vi "运维调试_五参数.vi"() -> ()   [LabVIEW 2016, in "斯坦道仪器.lvlib"]
uses:
  <vilib>/Utility/miscctls.llb/LVPointTypeDef.ctl
  PLC/PLC.lvlib
panel:
  in  "打开串口":bool
  in  "释放串口":bool
  out "数值 2":i32
  out "数值":i32
  in  "手动通电":bool
  out "多参数横条运行状态":T1(xcontrol)
  in  "数据区":i32(listbox)
  in  "探头选择":u16(ring)=9 items=["氨氮"=3, "水温"=9, "pH值"=10, "溶解氧"=11, "电导率"=12, "浊度"=13, "叶绿素a"=14, "藻密度"=15, "蓝绿藻"=16, "氧化还原电位"=17, "溶解氧%"=18, "盐度"=19]
  in  "测量数据区读取":bool
  in  "测量数据区":i32(listbox)
  in  "状态告警区读取":bool
  in  "状态告警区":i32(listbox)
  in  "自动校准":bool
  in  "读取KB":bool
  in  "写入KB":bool
  out "B":dbl caption="校准值B:"
  out "K":dbl caption="校准值K:"
  in  "校准区探头选择":u16(ring)=9 items=["氨氮"=3, "水温"=9, "pH值"=10, "溶解氧"=11, "电导率"=12, "浊度"=13, "叶绿素a"=14, "藻密度"=15, "蓝绿藻"=16, "氧化还原电位"=17, "溶解氧%"=18, "盐度"=19]
  in  "停止测量(单探)":bool
  in  "启动测量(单探)":bool
  in  "控制命令区探头选择":u16(ring)=9 items=["氨氮"=3, "水温"=9, "pH值"=10, "溶解氧"=11, "电导率"=12, "浊度"=13, "叶绿素a"=14, "藻密度"=15, "蓝绿藻"=16, "氧化还原电位"=17, "溶解氧%"=18, "盐度"=19]
  in  "同步时间":bool
  in  "初始化(清洗)":bool
  in  "停止测量(全部)":bool
  in  "启动测量(全部)":bool
  in  "关键参数区读取":bool
  in  "关键参数区":i32(listbox)
  in  "传感器参数读取":bool
  in  "传感器区":i32(listbox)
  in  "返回":bool
  in  "设置":bool
  out "运行状态":string
  out "开机状态":bool
  in  "停止":bool
  in  "手动启动":bool
  out "集成报警信息":string
  # "控制命令区"
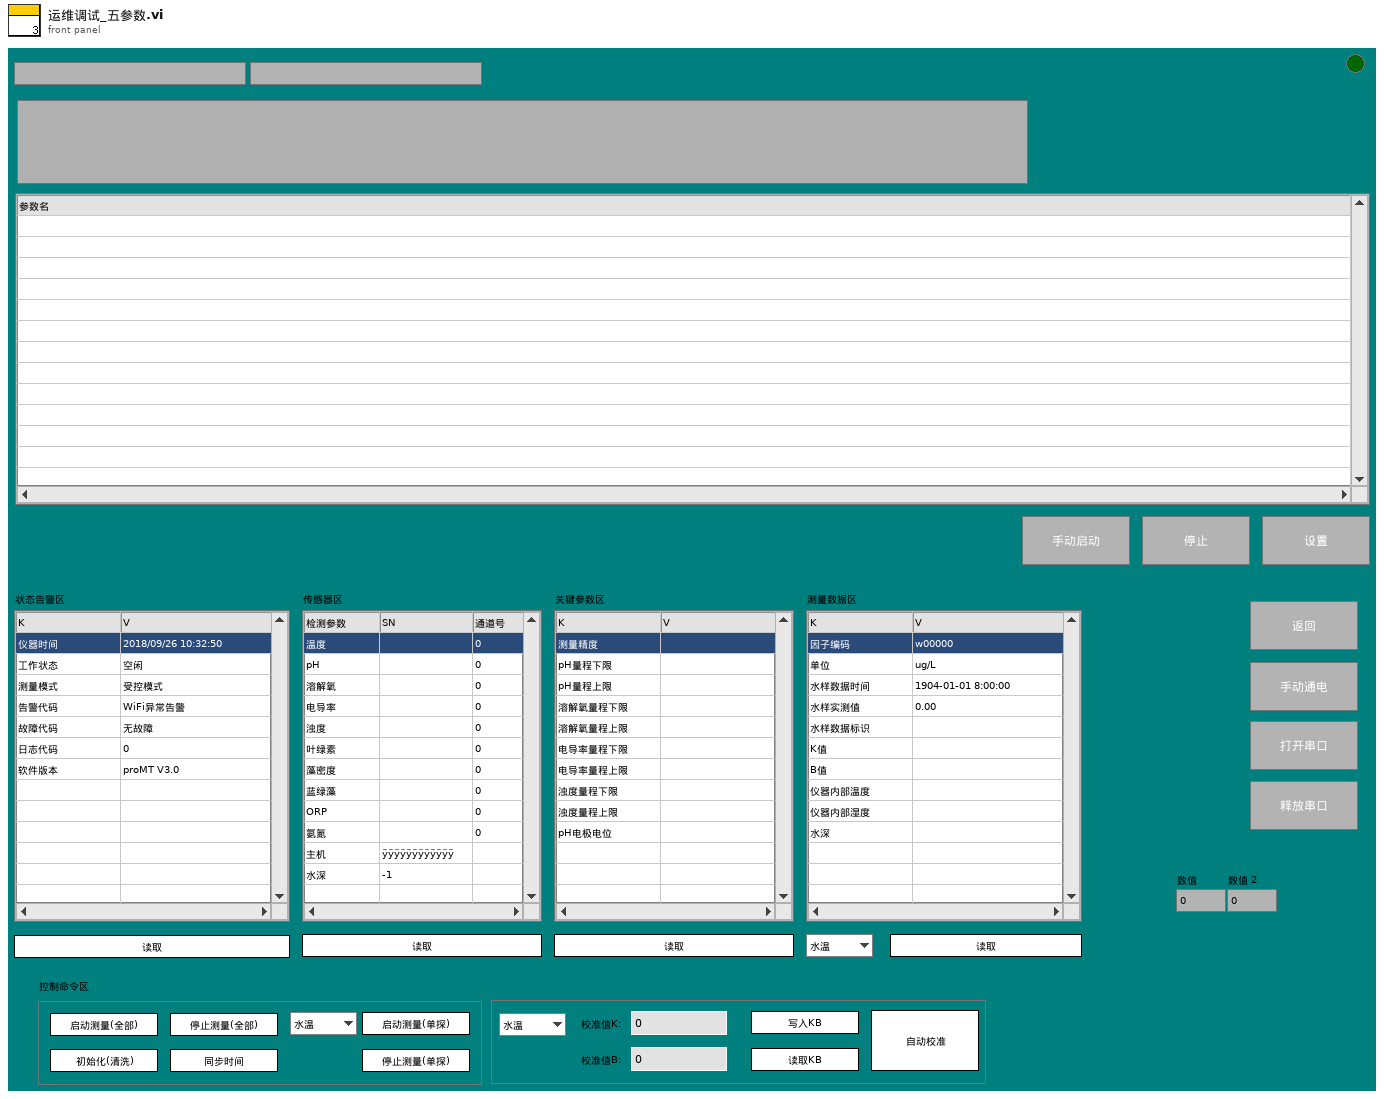
[diagram p1: front panel]
types:
  T1 = cluster{"系统时间":timestamp, "工作状态":u16, "测量模式":u16, "告警代码":enum16{"无告警", "缺试剂告警", "缺水样告警", "缺蒸馏水告警", "缺标液告警", "仪表漏液告警", "标定异常告警", "超量程告警", "加热异常", "低试剂预警", "超上限告警", "超下限告警", "仪表内部其他异常", "滴定异常告警", "电极异常告警", "量程切换告警", "参数设置告警", "PH电极电位异常", "电导率电极异常", "浊度光度异常", "溶解氧电极异常", "溶解氧光强异常", "温度异常告警", "PH异常告警", "溶解氧异常告警", "电导率异常告警", "浊度异常告警", "叶绿素异常告警", "藻密度异常告警", "蓝绿藻异常告警", "ORP异常告警", "氨氮异常告警", "清洁刷异常告警", "SD卡异常告警", "蓝牙异常告警", "Wifi异常告警", "流程异常告警"}, "故障代码":enum16{"无故障", "电机故障", "温度故障", "通讯故障", "滴定故障"}, "日志代码":u16, "软件版本":string}
  T2 = typedef "LVPointTypeDef.ctl" = cluster{"Horizontal":i16, "Vertical":i16}
  T3 = cluster{"时间标识":timestamp, "设备":string, "日志信息":string}
  T4 = enum16{"无告警", "缺试剂告警", "缺水样告警", "缺蒸馏水告警", "缺标液告警", "仪表漏液告警", "标定异常告警", "超量程告警", "加热异常", "低试剂预警", "超上限告警", "超下限告警", "仪表内部其他异常", "滴定异常告警", "电极异常告警", "量程切换告警", "参数设置告警", "PH电极电位异常", "电导率电极异常", "浊度光度异常", "溶解氧电极异常", "溶解氧光强异常", "温度异常告警", "PH异常告警", "溶解氧异常告警", "电导率异常告警", "浊度异常告警", "叶绿素异常告警", "藻密度异常告警", "蓝绿藻异常告警", "ORP异常告警", "氨氮异常告警", "清洁刷异常告警", "SD卡异常告警", "蓝牙异常告警", "Wifi异常告警", "流程异常告警"}
  T5 = cluster{"WORD[0]":u16, "WORD[1]":u16, "WORD[2]":u16, "WORD[3]":u16, "WORD[4]":u16, "WORD[5]":u16, "WORD[6]":u16, "WORD[7]":u16, "WORD[8]":u16, "WORD[9]":u16}
  T6 = cluster{"因子编码":string, "单位":string, "标样参考值":sgl, "水样数据时间":timestamp, "水样实测值":sgl, "水样数据标识":string, "K":sgl, "B":sgl, "T":sgl, "H":sgl, "水深":sgl}
  T7 = enum8{"Enabled", "Disabled", "Disabled and Grayed Out"}
  T8 = cluster{"测量模式":enum16{"待机", "水样测试", "标样核查", "零点核查", "跨度核查", "空白测试", "平行样测试", "加标回收", "空白校准", "标样校准", "初始化（清洗）"}, "数据标记表":string, "测量时间":dbl}
  T9 = cluster{"starting address":u16, "holding register value":u16}
  T10 = enum16{"idle", "init", "读状态", "读参数", "多个写入", "单个写入", "线圈写入"}
  T11 = enum32{"Bad", "Idle", "Run top level", "Running"}
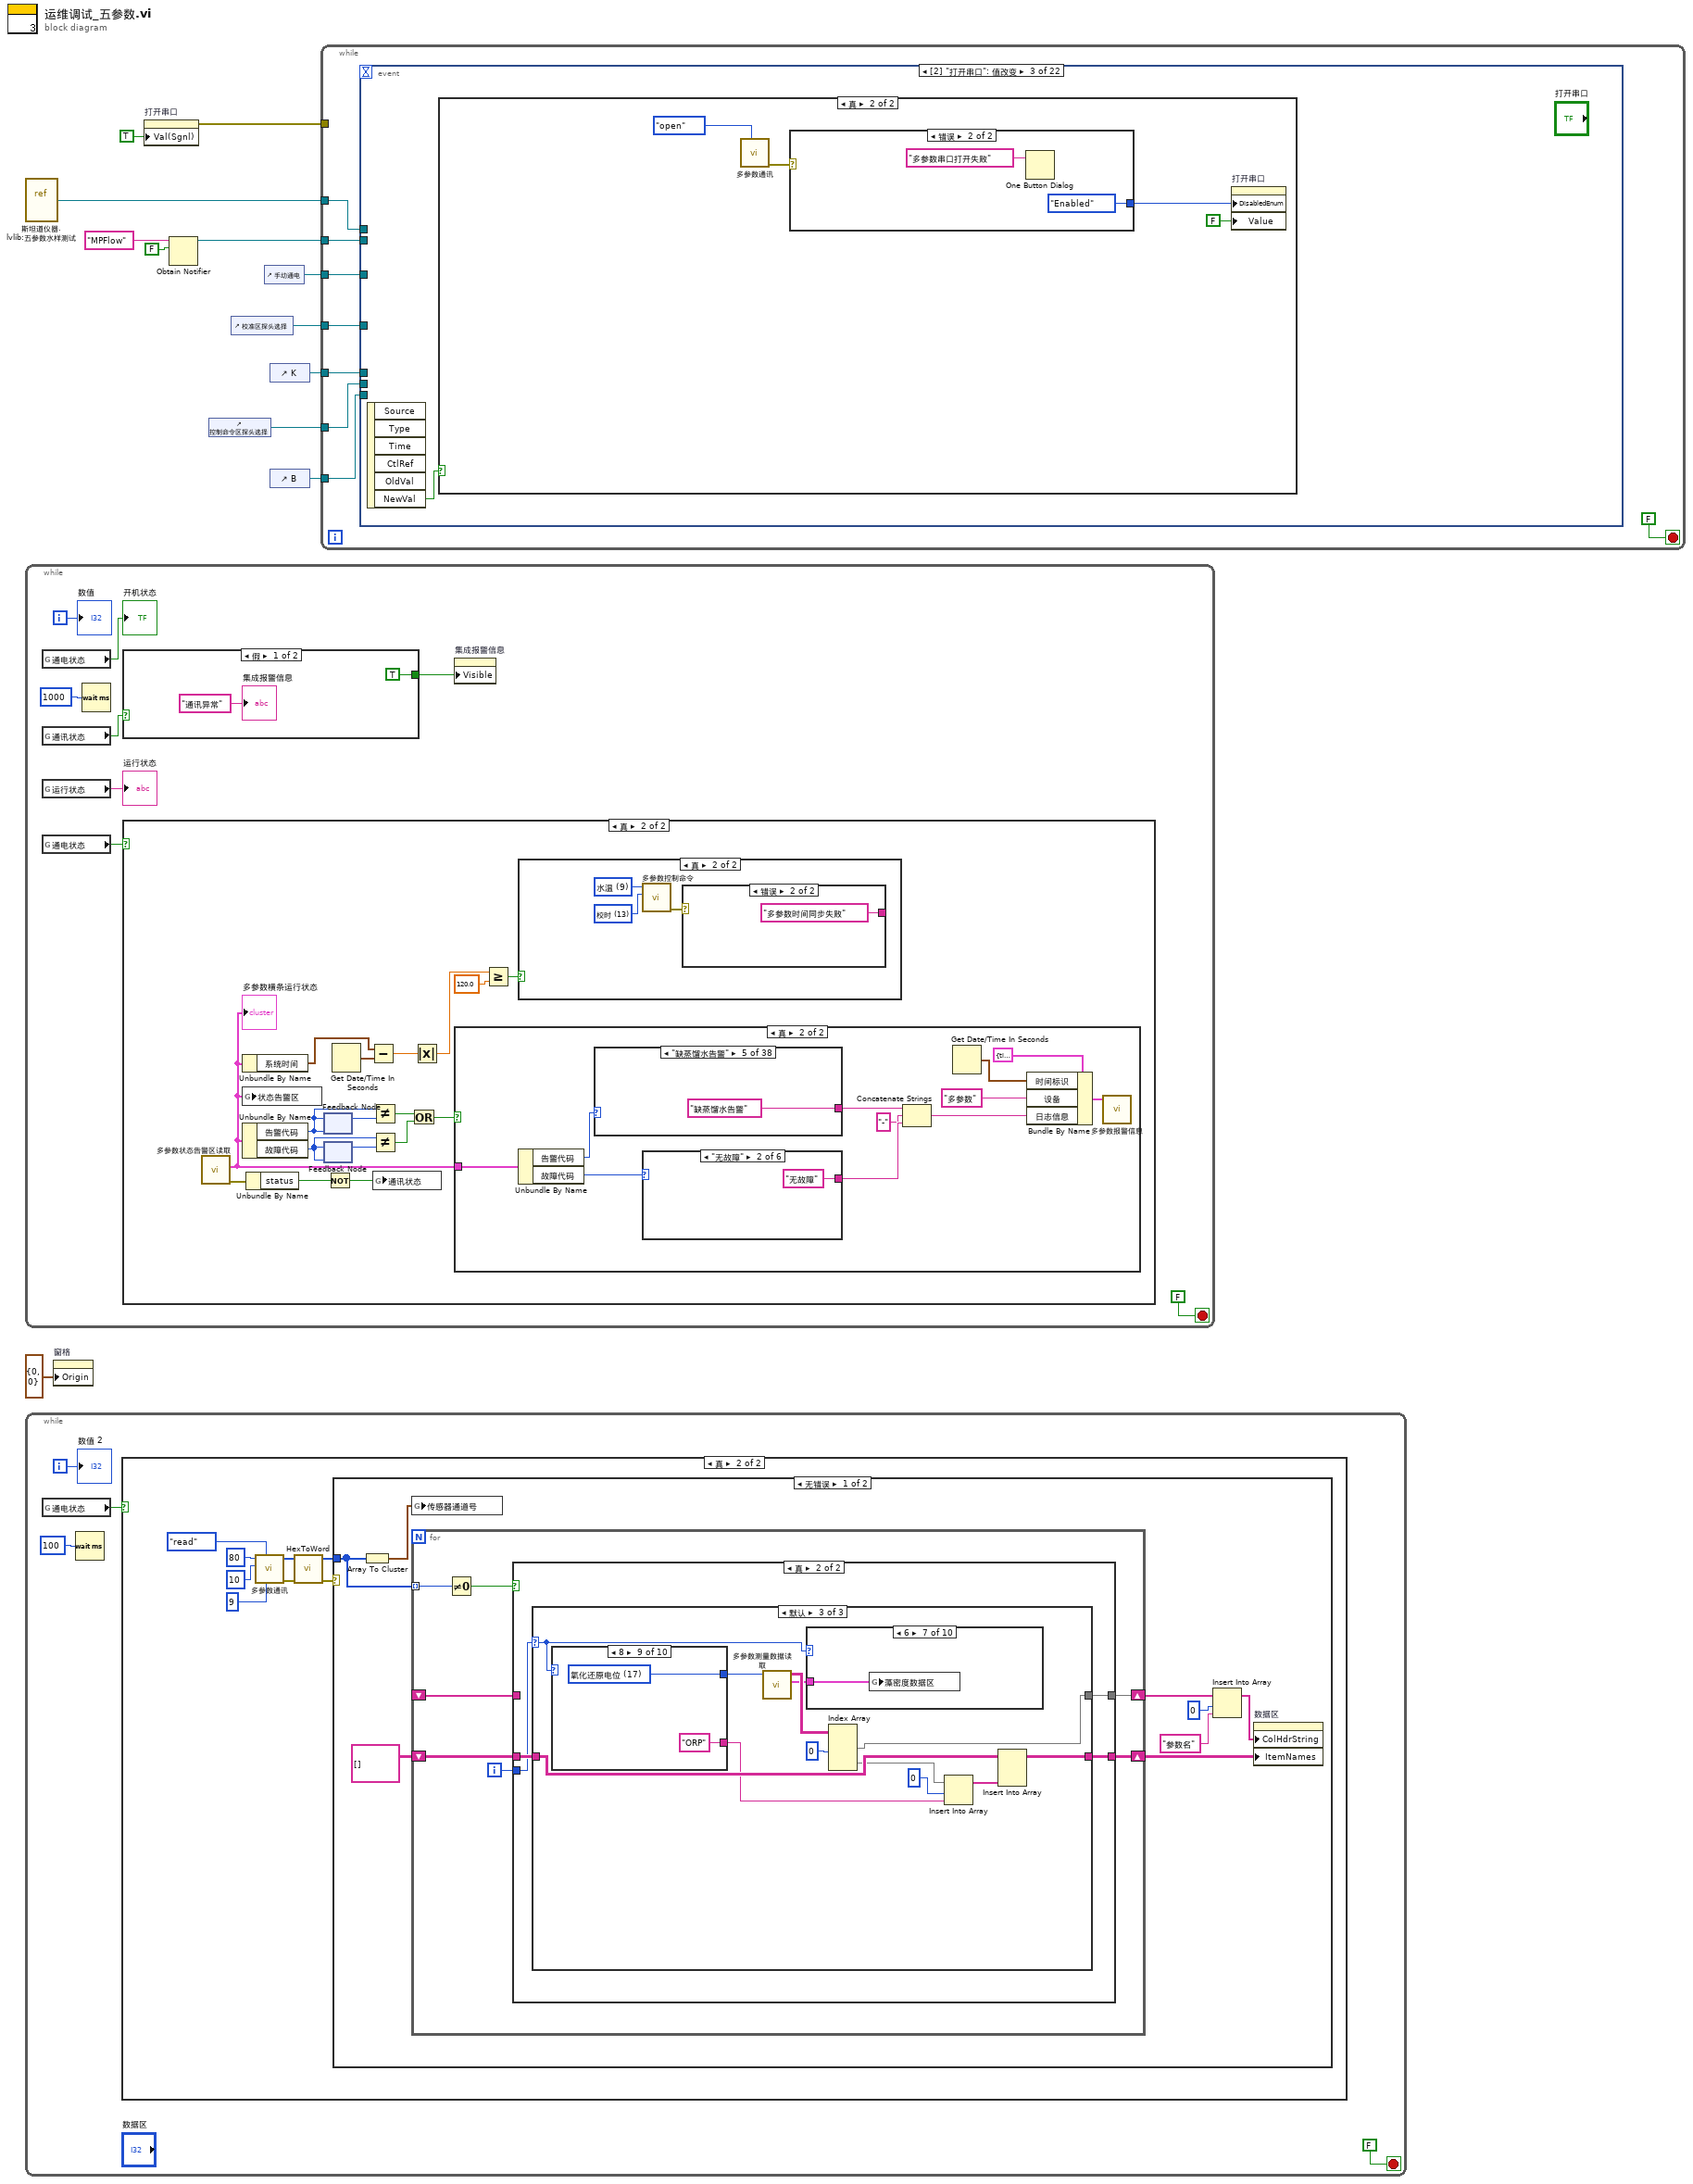
[diagram p0: block diagram]
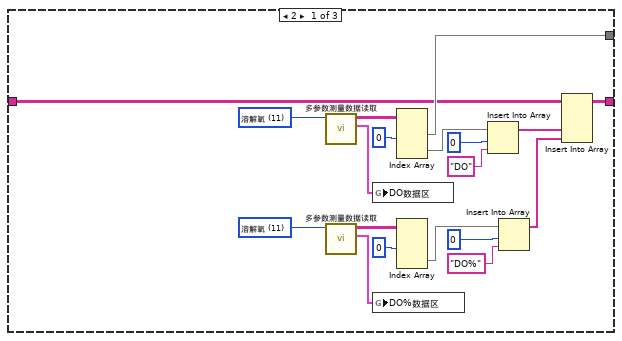
[diagram p4: hidden frame]
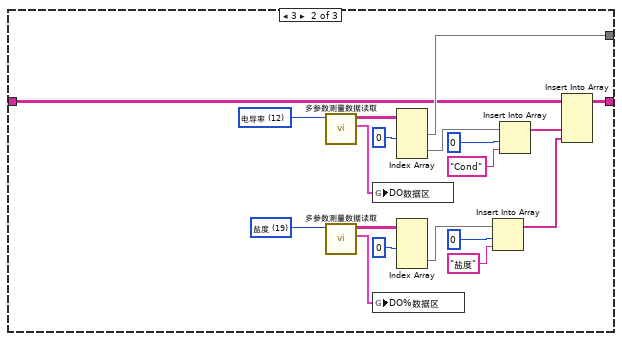
[diagram p5: hidden frame]
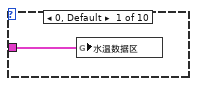
[diagram p6: hidden frame]
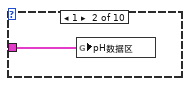
[diagram p7: hidden frame]
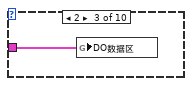
[diagram p8: hidden frame]
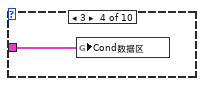
[diagram p9: hidden frame]
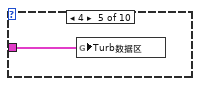
[diagram p10: hidden frame]
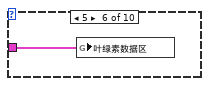
[diagram p11: hidden frame]
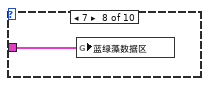
[diagram p12: hidden frame]
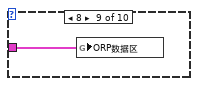
[diagram p13: hidden frame]
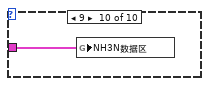
[diagram p14: hidden frame]
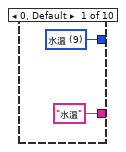
[diagram p15: hidden frame]
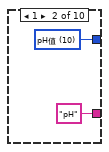
[diagram p16: hidden frame]
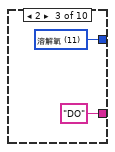
[diagram p17: hidden frame]
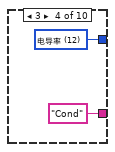
[diagram p18: hidden frame]
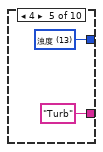
[diagram p19: hidden frame]
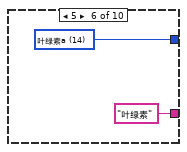
[diagram p20: hidden frame]
diagram:
  n1 = vi-ref "斯坦道仪器.lvlib:五参数水样测试.vi"() -> (w9:refnum<vi>)
  n2 = while {
    i -> [w13]
    stop <- FALSE stop-if-true
    n3 = global read "多参数全局变量.vi" "通电状态"() -> (→"开机状态":bool)
    n4 = global read "多参数全局变量.vi" "通讯状态"() -> (w18:bool)
    n5 = global read "多参数全局变量.vi" "运行状态"() -> (→"运行状态":string)
    n6 = global read "多参数全局变量.vi" "通电状态"() -> (w14:bool)
    n7 = Wait (ms)(milliseconds to wait=u32 1000 ("等待时间（毫秒）")) -> ()  [unwired: 1 out]
    n8 = case shown="假" w18 {
      tunnel: [TRUE ("可见") _] -> w17
      frame False {
        "集成报警信息" <- "通讯异常" ("集成报警信息")
      }
      frame True {
      }
    }
    n9 = case shown="真" w14 {
      frame False {
      }
      frame True {
        n10 = call "多参数状态告警区读取.vi"() -> ("error out"=w30:errorcluster, "状态告警块"=w27:T1)  [unwired: 9 in, 1 out]
        "多参数横条运行状态" <- w27
        n11 = Unbundle By Name(w27) -> ("系统时间"=w26:timestamp)
        n12 = global write "多参数全局变量.vi" "状态告警区"(w27) -> ()
        n13 = Unbundle By Name(w27) -> ("告警代码"=w36:T4, "故障代码"=w34:enum16{"无故障", "电机故障", "温度故障", "通讯故障", "滴定故障"})
        n14 = Unbundle By Name(w30) -> ("status"=w29:bool)
        n15 = feedback #1(w36) -> (w37:T4)
        n16 = feedback-in #1(w36) -> ()
        n17 = feedback #2(w34) -> (w35:enum16{"无故障", "电机故障", "温度故障", "通讯故障", "滴定故障"})
        n18 = feedback-in #2(w34) -> ()
        n19 = Not(x=w29) -> (.not. x?=w28:bool)
        n20 = Get Date/Time In Seconds() -> (seconds since 1Jan1904=w25:timestamp)
        n21 = Subtract(x=w26, y=w25) -> (x-y=w24:dbl)
        n22 = Not Equal?(x=w36, y=w37) -> (x != y?=w32:bool)
        n23 = Not Equal?(x=w34, y=w35) -> (x != y?=w33:bool)
        n24 = global write "多参数全局变量.vi" "通讯状态"(w28) -> ()
        n25 = Or(x=w32, y=w33) -> (x .or. y?=w31:bool)
        n26 = Absolute Value(x=w24) -> (abs(x)=w23:dbl)
        n27 = case shown="真" w31 {
          tunnel: w27 -> [_ w53]
          frame False {
          }
          frame True {
            n28 = Unbundle By Name(w53) -> ("告警代码"=w52:T4, "故障代码"=w51:enum16{"无故障", "电机故障", "温度故障", "通讯故障", "滴定故障"})
            n29 = case shown="\"缺蒸馏水告警\"" w52 {
              selector: w52 -> [w64 _ _ _ _ _ _ _ _ _ _ _ _ _ _ _ _ _ _ _ _ _ _ _ _ _ _ _ _ _ _ _ _ _ _ _ _ _]
              tunnel: [w63 "无告警" "缺试剂告警" "缺水样告警" "缺蒸馏水告警" "缺标液告警" "仪表漏液告警" "标定异常告警" "超量程告警" "加热异常" "低试剂预警" "超上限告警" "超下限告警" "仪表内部其他异常" "滴定异常告警" "电极异常告警" "量程切换告警" "参数设置告警" "PH电极电位异常" "电导率电极异常" "浊度光度异常" "溶解氧电极异常" "溶解氧光强异常" "温度异常告警" "PH异常告警" "溶解氧异常告警" "电导率异常告警" "浊度异常告警" "叶绿素异常告警" "藻密度异常告警" "蓝绿藻异常告警" "ORP异常告警" "氨氮异常告警" "清洁刷异常告警" "SD卡异常告警" "蓝牙异常告警" "WiFi异常告警" "流程异常告警"] -> w50
              frame Default {
                n30 = Format Into String(format string="%d" ("格式字符串"), initial string="未知" ("工作状态"), w64) -> (resulting string=w63:string)  [unwired: 1 in, 1 out]
              }
              frame "无告警" {
              }
              frame "缺试剂告警" {
              }
              frame "缺水样告警" {
              }
              frame "缺蒸馏水告警" {
              }
              frame "缺标液告警" {
              }
              frame "仪表漏液告警" {
              }
              frame "标定异常告警" {
              }
              frame "超量程告警" {
              }
              frame "加热异常" {
              }
              frame "低试剂预警" {
              }
              frame "超上限告警" {
              }
              frame "超下限告警" {
              }
              frame "仪表内部其他异常" {
              }
              frame "滴定异常告警" {
              }
              frame "电极异常告警" {
              }
              frame "量程切换告警" {
              }
              frame "参数设置告警" {
              }
              frame "PH电极电位异常" {
              }
              frame "电导率电极异常" {
              }
              frame "浊度光度异常" {
              }
              frame "溶解氧电极异常" {
              }
              frame "溶解氧光强异常" {
              }
              frame "温度异常告警" {
              }
              frame "PH异常告警" {
              }
              frame "溶解氧异常告警" {
              }
              frame "电导率异常告警" {
              }
              frame "浊度异常告警" {
              }
              frame "叶绿素异常告警" {
              }
              frame "藻密度异常告警" {
              }
              frame "蓝绿藻异常告警" {
              }
              frame "ORP异常告警" {
              }
              frame "氨氮异常告警" {
              }
              frame "清洁刷异常告警" {
              }
              frame "SD卡异常告警" {
              }
              frame "蓝牙异常告警" {
              }
              frame "Wifi异常告警" {
              }
              frame "流程异常告警" {
              }
            }
            n31 = case shown="\"无故障\"" w51 {
              selector: w51 -> [w55 _ _ _ _ _]
              tunnel: [w54 "无故障" "电机故障" "温度故障" "通讯故障" "滴定故障"] -> w49
              frame Default {
                n32 = Format Into String(format string="%d" ("格式字符串"), initial string="未知" ("工作状态"), w55) -> (resulting string=w54:string)  [unwired: 1 in, 1 out]
              }
              frame "无故障" {
              }
              frame "电机故障" {
              }
              frame "温度故障" {
              }
              frame "通讯故障" {
              }
              frame "滴定故障" {
              }
            }
            n33 = Concatenate Strings(w50, "-" ("字符串"), w49) -> (w45:string)
            n34 = Get Date/Time In Seconds() -> (seconds since 1Jan1904=w44:timestamp)
            n35 = Bundle By Name(cluster=T3 {"时间标识"=timestamp(0 s since 1904-01-01), "设备"="", "日志信息"=""} ("data in"), "时间标识"=w44, "设备"="多参数", "日志信息"=w45) -> (w46:T3)
            n36 = call "多参数报警信息.vi"("data in"=w46) -> ()  [unwired: 10 in, 1 out]
          }
        }
        n37 = Greater Or Equal?(x=w23, y=120.0) -> (x >= y?=w22:bool)
        n38 = case shown="真" w22 {
          frame False {
          }
          frame True {
            w38 = u16 13 items=["启动测量（全部）"=1, "初始化（清洗）"=10, "停止测量（全部）"=11, "校时"=13, "启动测量（单个传感器）"=19, "停止测量（单个传感器）"=20] ("控制命令")
            w39 = u16 9 items=["氨氮"=3, "水温"=9, "pH值"=10, "溶解氧"=11, "电导率"=12, "浊度"=13, "叶绿素a"=14, "藻密度"=15, "蓝绿藻"=16, "氧化还原电位"=17, "溶解氧%"=18, "盐度"=19] ("站号")
            n39 = call "多参数控制命令.vi"("控制命令"=w38, "站号"=w39) -> ("error out"=w40:errorcluster)  [unwired: 9 in]
            n40 = case shown="错误" w40 {
              tunnel: ["多参数时间同步成功" ("消息") "多参数时间同步失败" ("消息")] -> _
              frame No Error {
              }
              frame Error {
              }
            }
          }
        }
      }
    }
    n41 = property on="集成报警信息" class="Str"("Visible"=w17) -> ()  [unwired: 2 in, 2 out]
    "数值" <- w13
  }
  n42 = while {
    i -> [w106]
    stop <- FALSE stop-if-true
    n43 = global read "多参数全局变量.vi" "通电状态"() -> (w107:bool)
    n44 = Wait (ms)(milliseconds to wait=u32 100 ("等待时间（毫秒）")) -> ()  [unwired: 1 out]
    n45 = case shown="真" w107 {
      frame False {
      }
      frame True {
        n46 = call "多参数通讯.vi"("Slave ID"=u8 9, "STEP"=enum16{"open", "read", "write", "close"}."read", "quantity"=u16 10, "starting address"=u16 80) -> ("error out"=w112:errorcluster, "Registers"=w113:u16[])  [unwired: 5 in, 1 out]
        n47 = call "HexToWord.vi"("数组"=w113) -> ("WORD"=w116:u16[])  [unwired: 10 in]
        n48 = case shown="无错误" w112 {
          tunnel: w116 -> [w117 _]
          frame No Error {
            n49 = Array To Cluster(array=w117) -> (cluster=w118:T5)
            n50 = global write "多参数全局变量.vi" "传感器通道号"(w118) -> ()
            n51 = for {
              tunnel: w117 -> [w130] mode=indexing
              shift-right: [w128] -> w122
              shift-left: _ -> [w127]
              shift-right: [w125] -> w123
              shift-left: string[][] [] ("子数组") -> [w126]
              i -> [w131]
              n52 = Not Equal To 0?(x=w130) -> (x != 0?=w129:bool)
              n53 = case shown="真" w129 {
                tunnel: w131 -> [_ w134]
                tunnel: [w133 w137] -> w128
                tunnel: w127 -> [w133 _]
                tunnel: w126 -> [w132 w136]
                tunnel: [w132 w135] -> w125
                frame False {
                }
                frame True {
                  n54 = case shown="默认" w134 {
                    selector: w134 -> [_ _ w176]
                    tunnel: [w146 w165 w184] -> w137
                    tunnel: w136 -> [w142 w161 w183]
                    tunnel: [w145 w164 w182] -> w135
                    frame 2 {
                      w140 = u16 11 items=["氨氮"=3, "水温"=9, "pH值"=10, "溶解氧"=11, "电导率"=12, "浊度"=13, "叶绿素a"=14, "藻密度"=15, "蓝绿藻"=16, "氧化还原电位"=17, "溶解氧%"=18, "盐度"=19] ("探头选择")
                      w141 = u16 11 items=["氨氮"=3, "水温"=9, "pH值"=10, "溶解氧"=11, "电导率"=12, "浊度"=13, "叶绿素a"=14, "藻密度"=15, "蓝绿藻"=16, "氧化还原电位"=17, "溶解氧%"=18, "盐度"=19] ("探头选择")
                      n55 = call "多参数测量数据读取.vi"("探头选择"=w141) -> ("测量数据块"=w139:T6, "添加的数组"=w144:string[][])  [unwired: 8 in, 1 out]
                      n56 = call "多参数测量数据读取.vi"("探头选择"=w140) -> ("测量数据块"=w138:T6, "添加的数组"=w143:string[][])  [unwired: 8 in, 1 out]
                      n57 = global write "多参数全局变量.vi" "DO数据区"(w139) -> ()
                      n58 = global write "多参数全局变量.vi" "DO%数据区"(w138) -> ()
                      n59 = Index Array(array=w144, index (col) #1=0 ("禁用的索引 (列)")) -> (element #1=w146:string[], element #2=w155:string[])  [unwired: 3 in]
                      n60 = Index Array(array=w143, index (col) #1=0 ("禁用的索引 (列)")) -> (element #2=w151:string[])  [unwired: 3 in, 1 out]
                      n61 = Insert Into Array(array=w155, index=0 ("索引"), new element="DO") -> (w153:string[])
                      n62 = Insert Into Array(array=w151, index=0 ("索引"), new element="DO%") -> (w150:string[])
                      n63 = Insert Into Array(array=w142, new element #1=w153, new element #2=w150) -> (w145:string[][])  [unwired: 2 in]
                    }
                    frame 3 {
                      w159 = u16 19 items=["氨氮"=3, "水温"=9, "pH值"=10, "溶解氧"=11, "电导率"=12, "浊度"=13, "叶绿素a"=14, "藻密度"=15, "蓝绿藻"=16, "氧化还原电位"=17, "溶解氧%"=18, "盐度"=19] ("探头选择")
                      w160 = u16 12 items=["氨氮"=3, "水温"=9, "pH值"=10, "溶解氧"=11, "电导率"=12, "浊度"=13, "叶绿素a"=14, "藻密度"=15, "蓝绿藻"=16, "氧化还原电位"=17, "溶解氧%"=18, "盐度"=19] ("探头选择")
                      n64 = call "多参数测量数据读取.vi"("探头选择"=w160) -> ("测量数据块"=w158:T6, "添加的数组"=w163:string[][])  [unwired: 8 in, 1 out]
                      n65 = call "多参数测量数据读取.vi"("探头选择"=w159) -> ("测量数据块"=w157:T6, "添加的数组"=w162:string[][])  [unwired: 8 in, 1 out]
                      n66 = global write "多参数全局变量.vi" "DO数据区"(w158) -> ()
                      n67 = global write "多参数全局变量.vi" "DO%数据区"(w157) -> ()
                      n68 = Index Array(array=w163, index (col) #1=0 ("禁用的索引 (列)")) -> (element #1=w165:string[], element #2=w174:string[])  [unwired: 3 in]
                      n69 = Index Array(array=w162, index (col) #1=0 ("禁用的索引 (列)")) -> (element #2=w170:string[])  [unwired: 3 in, 1 out]
                      n70 = Insert Into Array(array=w170, index=0 ("索引"), new element="盐度") -> (w169:string[])
                      n71 = Insert Into Array(array=w174, index=0 ("索引"), new element="Cond") -> (w172:string[])
                      n72 = Insert Into Array(array=w161, new element #1=w172, new element #2=w169) -> (w164:string[][])  [unwired: 2 in]
                    }
                    frame Default {
                      n73 = case shown="8" w176 {
                        tunnel: [w199 w201 w203 w205 w207 w209 w211 w213 w215 w217] -> w187
                        tunnel: ["水温" "pH" "DO" "Cond" "Turb" "叶绿素" "藻密度" "蓝绿藻" "ORP" "氨氮"] -> w180
                        frame 0, Default {
                          w199 = u16 9 items=["氨氮"=3, "水温"=9, "pH值"=10, "溶解氧"=11, "电导率"=12, "浊度"=13, "叶绿素a"=14, "藻密度"=15, "蓝绿藻"=16, "氧化还原电位"=17, "溶解氧%"=18, "盐度"=19] ("探头选择")
                        }
                        frame 1 {
                          w201 = u16 10 items=["氨氮"=3, "水温"=9, "pH值"=10, "溶解氧"=11, "电导率"=12, "浊度"=13, "叶绿素a"=14, "藻密度"=15, "蓝绿藻"=16, "氧化还原电位"=17, "溶解氧%"=18, "盐度"=19] ("探头选择")
                        }
                        frame 2 {
                          w203 = u16 11 items=["氨氮"=3, "水温"=9, "pH值"=10, "溶解氧"=11, "电导率"=12, "浊度"=13, "叶绿素a"=14, "藻密度"=15, "蓝绿藻"=16, "氧化还原电位"=17, "溶解氧%"=18, "盐度"=19] ("探头选择")
                        }
                        frame 3 {
                          w205 = u16 12 items=["氨氮"=3, "水温"=9, "pH值"=10, "溶解氧"=11, "电导率"=12, "浊度"=13, "叶绿素a"=14, "藻密度"=15, "蓝绿藻"=16, "氧化还原电位"=17, "溶解氧%"=18, "盐度"=19] ("探头选择")
                        }
                        frame 4 {
                          w207 = u16 13 items=["氨氮"=3, "水温"=9, "pH值"=10, "溶解氧"=11, "电导率"=12, "浊度"=13, "叶绿素a"=14, "藻密度"=15, "蓝绿藻"=16, "氧化还原电位"=17, "溶解氧%"=18, "盐度"=19] ("探头选择")
                        }
                        frame 5 {
                          w209 = u16 14 items=["氨氮"=3, "水温"=9, "pH值"=10, "溶解氧"=11, "电导率"=12, "浊度"=13, "叶绿素a"=14, "藻密度"=15, "蓝绿藻"=16, "氧化还原电位"=17, "溶解氧%"=18, "盐度"=19] ("探头选择")
                        }
                        frame 6 {
                          w211 = u16 15 items=["氨氮"=3, "水温"=9, "pH值"=10, "溶解氧"=11, "电导率"=12, "浊度"=13, "叶绿素a"=14, "藻密度"=15, "蓝绿藻"=16, "氧化还原电位"=17, "溶解氧%"=18, "盐度"=19] ("探头选择")
                        }
                        frame 7 {
                          w213 = u16 16 items=["氨氮"=3, "水温"=9, "pH值"=10, "溶解氧"=11, "电导率"=12, "浊度"=13, "叶绿素a"=14, "藻密度"=15, "蓝绿藻"=16, "氧化还原电位"=17, "溶解氧%"=18, "盐度"=19] ("探头选择")
                        }
                        frame 8 {
                          w215 = u16 17 items=["氨氮"=3, "水温"=9, "pH值"=10, "溶解氧"=11, "电导率"=12, "浊度"=13, "叶绿素a"=14, "藻密度"=15, "蓝绿藻"=16, "氧化还原电位"=17, "溶解氧%"=18, "盐度"=19] ("探头选择")
                        }
                        frame 9 {
                          w217 = u16 3 items=["氨氮"=3, "水温"=9, "pH值"=10, "溶解氧"=11, "电导率"=12, "浊度"=13, "叶绿素a"=14, "藻密度"=15, "蓝绿藻"=16, "氧化还原电位"=17, "溶解氧%"=18, "盐度"=19] ("探头选择")
                        }
                      }
                      n74 = call "多参数测量数据读取.vi"("探头选择"=w187) -> ("测量数据块"=w177:T6, "添加的数组"=w186:string[][])  [unwired: 8 in, 1 out]
                      n75 = case shown="6" w176 {
                        tunnel: w177 -> [w188 w189 w190 w191 w192 w193 w194 w195 w196 w197]
                        frame 0, Default {
                          n76 = global write "多参数全局变量.vi" "水温数据区"(w188) -> ()
                        }
                        frame 1 {
                          n77 = global write "多参数全局变量.vi" "pH数据区"(w189) -> ()
                        }
                        frame 2 {
                          n78 = global write "多参数全局变量.vi" "DO数据区"(w190) -> ()
                        }
                        frame 3 {
                          n79 = global write "多参数全局变量.vi" "Cond数据区"(w191) -> ()
                        }
                        frame 4 {
                          n80 = global write "多参数全局变量.vi" "Turb数据区"(w192) -> ()
                        }
                        frame 5 {
                          n81 = global write "多参数全局变量.vi" "叶绿素数据区"(w193) -> ()
                        }
                        frame 6 {
                          n82 = global write "多参数全局变量.vi" "藻密度数据区"(w194) -> ()
                        }
                        frame 7 {
                          n83 = global write "多参数全局变量.vi" "蓝绿藻数据区"(w195) -> ()
                        }
                        frame 8 {
                          n84 = global write "多参数全局变量.vi" "ORP数据区"(w196) -> ()
                        }
                        frame 9 {
                          n85 = global write "多参数全局变量.vi" "NH3N数据区"(w197) -> ()
                        }
                      }
                      n86 = Index Array(array=w186, index (col) #1=0 ("禁用的索引 (列)")) -> (element #1=w184:string[], element #2=w181:string[])  [unwired: 3 in]
                      n87 = Insert Into Array(array=w181, index=0 ("索引"), new element=w180) -> (w179:string[])
                      n88 = Insert Into Array(array=w183, new element=w179) -> (w182:string[][])  [unwired: 2 in]
                    }
                  }
                }
              }
            }
            n89 = Insert Into Array(array=w122, index=0 ("索引"), new element="参数名" ("新元素/子数组")) -> (w121:string[])
            n90 = property on="数据区" class="MCListbox (严格)"("ColHdrString"=w121, "ItemNames"=w123) -> ()  [unwired: 2 in, 2 out]
          }
          frame Error {
          }
        }
      }
    }
    "数值 2" <- w106
  }
  n91 = property on="窗格" class="Pane"("Origin"=T2 {"Horizontal"=0, "Vertical"=0} ("原点")) -> ()  [unwired: 2 in, 2 out]
  n92 = property on="打开串口" class="Bool (严格)"("Val(Sgnl)"=TRUE ("值(信号)")) -> (error out=w1:errorcluster)  [unwired: 2 in, 1 out]
  n93 = Obtain Notifier(name (unnamed)="MPFlow" ("名称（未命名）"), notification data type=FALSE) -> (notifier out=w8:refnum<notifier>)  [unwired: 2 in, 2 out]
  n94 = control-ref of="控制命令区探头选择"() -> (w7:refnum<vi>)
  n95 = control-ref of="校准区探头选择"() -> (w4:refnum<vi>)
  n96 = control-ref of="手动通电"() -> (w3:refnum<vi>)
  n97 = control-ref of="K"() -> (w6:refnum<vi>)
  n98 = control-ref of="B"() -> (w5:refnum<vi>)
  n99 = while {
    tunnel: w9 -> [w224]
    tunnel: w8 -> [w223]
    tunnel: w7 -> [w222]
    tunnel: w6 -> [w221]
    tunnel: w5 -> [w220]
    tunnel: w4 -> [w219]
    tunnel: w3 -> [w218]
    tunnel: w1 -> [_]
    stop <- FALSE stop-if-true
    n100 = event shown="[2] \"打开串口\": 值改变" {
      selector: _ -> [_ _ _ _ _ _ _ _ _ _ _ _ _ _ _ _ _ _ _ _ _ _]
      dyn-events: _ -> [_ _ _ _ _ _ _ _ _ _ _ _ _ _ _ _ _ _ _ _ _ _]
      timeout: _ -> [_ _ _ _ _ _ _ _ _ _ _ _ _ _ _ _ _ _ _ _ _ _]
      tunnel: w224 -> [_ _ _ w240 _ _ _ _ _ _ _ _ _ _ _ _ _ _ _ _ _ _]
      tunnel: w223 -> [_ _ _ _ w262 _ _ _ _ _ _ _ _ _ _ _ _ _ _ _ _ _]
      tunnel: w222 -> [_ _ _ _ _ _ _ _ _ _ _ _ _ _ _ w329 w340 _ _ _ _ _]
      tunnel: w221 -> [_ _ _ _ _ _ _ _ _ _ _ _ _ _ _ _ _ w351 _ _ _ _]
      tunnel: w220 -> [_ _ _ _ _ _ _ _ _ _ _ _ _ _ _ _ _ w353 _ _ _ _]
      tunnel: w219 -> [_ _ _ _ _ _ _ _ _ _ _ _ _ _ _ _ _ w355 _ w371 _ _]
      tunnel: w218 -> [_ _ _ _ _ _ _ w270 w275 w280 w286 w291 w300 w309 w318 w327 w338 w349 _ w369 w381 _]
      event Timeout {
        n101 = event-data() -> ()  [unwired: 1 in, 3 out]
      }
      event "释放串口": Value Change {
        n102 = event-data() -> ("NewVal"=w226:bool)  [unwired: 1 in, 5 out]
        n103 = case shown="真" w226 {
          frame False {
          }
          frame True {
            n104 = call "多参数通讯.vi"("STEP"=enum16{"open", "read", "write", "close"}."close") -> ("error out"=w227:errorcluster)  [unwired: 8 in, 2 out]
            n105 = case shown="无错误" w227 {
              frame No Error {
                n106 = property on="打开串口" class="Bool (严格)"("DisabledEnum"=T7."Enabled" ("禁用")) -> ()  [unwired: 2 in, 2 out]
              }
              frame Error {
              }
            }
          }
        }
      }
      event "打开串口": Value Change {
        n107 = event-data() -> ("NewVal"=w230:bool)  [unwired: 1 in, 5 out]
        n108 = case shown="真" w230 {
          frame False {
          }
          frame True {
            n109 = call "多参数通讯.vi"("STEP"=enum16{"open", "read", "write", "close"}."open") -> ("error out"=w231:errorcluster)  [unwired: 8 in, 2 out]
            n110 = case shown="错误" w231 {
              tunnel: [T7."Disabled and Grayed Out" ("禁用") T7."Enabled" ("禁用")] -> w233
              frame No Error {
              }
              frame Error {
                n111 = One Button Dialog(message="多参数串口打开失败" ("消息")) -> ()  [unwired: 1 in, 1 out]
              }
            }
            n112 = property on="打开串口" class="Bool (严格)"("DisabledEnum"=w233, "Value"=FALSE ("打开串口")) -> ()  [unwired: 2 in, 2 out]
          }
        }
      }
      event "手动启动": Value Change {
        n113 = event-data() -> ()  [unwired: 1 in, 6 out]
        n114 = call "多参数启动参数对话框.vi"() -> ("确认"=w239:bool, "测量时间"=w238:dbl)  [unwired: 10 in]
        n115 = case shown="真" w239 {
          tunnel: w240 -> [_ w242]
          tunnel: w238 -> [_ w241]
          frame False {
          }
          frame True {
            n116 = property class="VI"(reference=w242) -> ("Name"=w246:string, "Exec.State"=w244:T11)  [unwired: 1 in, 2 out]
            n117 = Open VI Reference(type specifier VI Refnum (for type only)=refnum<vi> refnum ("类型说明符VI引用句柄（仅用于类型）"), vi path=w246, options=128 ("选项")) -> (vi reference=w245:refnum<vi>)  [unwired: 3 in, 1 out]
            n118 = case shown="\"Idle\"" w244 {
              tunnel: w245 -> [w250 w257]
              tunnel: [w250 w256] -> w243
              tunnel: w241 -> [_ w251]
              frame "Bad", Default {
                n119 = One Button Dialog(message="仪器已经启动，无需重复启动" ("消息")) -> ()  [unwired: 1 in, 1 out]
              }
              frame "Idle" {
                n120 = global read "系统变量.vi" "运行模式"() -> (w253:enum16{"维护模式", "常规模式", "应急模式", "质控模式"})
                n121 = case shown="\"常规模式\", 默认" w253 {
                  tunnel: ["M" ("数据标记表") "hd" ("数据标记表")] -> w252
                  frame "维护模式" {
                  }
                  frame "常规模式", Default {
                  }
                }
                n122 = Bundle By Name(cluster=T8 {"测量模式"=enum."水样测试", "数据标记表"="", "测量时间"=0.0} ("启动参数"), "数据标记表"=w252, "测量时间"=w251) -> (w254:T8)
                n123 = call-by-ref "开始异步调用"(reference=w257, "启动参数"=w254) -> (reference out=w256:refnum<vi>)  [unwired: 12 in, 1 out]
              }
            }
            n124 = Close Reference(reference=w243) -> ()  [unwired: 1 in, 1 out]
          }
        }
      }
      event "停止": Value Change {
        n125 = event-data() -> ()  [unwired: 1 in, 6 out]
        n126 = Two Button Dialog(message="请再一次确认是否停止测量" ("消息")) -> (T button?=w260:bool)  [unwired: 2 in]
        n127 = case shown="真" w260 {
          tunnel: w262 -> [_ w265]
          frame False {
          }
          frame True {
            w263 = u16 11 items=["启动测量（全部）"=1, "初始化（清洗）"=10, "停止测量（全部）"=11, "校时"=13, "启动测量（单个传感器）"=19, "停止测量（单个传感器）"=20] ("控制命令")
            w264 = u16 10 items=["氨氮"=3, "水温"=9, "pH值"=10, "溶解氧"=11, "电导率"=12, "浊度"=13, "叶绿素a"=14, "藻密度"=15, "蓝绿藻"=16, "氧化还原电位"=17, "溶解氧%"=18, "盐度"=19] ("站号")
            n128 = Send Notification(notification=TRUE ("通知"), notifier=w265) -> ()  [unwired: 1 in, 2 out]
            n129 = call "多参数控制命令.vi"("控制命令"=w263, "站号"=w264) -> ()  [unwired: 9 in, 1 out]
          }
        }
      }
      event "设置": Value Change {
        n130 = event-data() -> ()  [unwired: 1 in, 6 out]
        n131 = property on="窗格" class="Pane"("Origin"=T2 {"Horizontal"=0, "Vertical"=528} ("原点")) -> ()  [unwired: 2 in, 2 out]
      }
      event "返回": Value Change {
        n132 = event-data() -> ()  [unwired: 1 in, 6 out]
        n133 = property on="窗格" class="Pane"("Origin"=T2 {"Horizontal"=0, "Vertical"=0} ("原点")) -> ()  [unwired: 2 in, 2 out]
      }
      event "传感器参数读取": Value Change {
        n134 = event-data() -> ()  [unwired: 1 in, 6 out]
        n135 = property class="Bool (严格)"(reference=w270) -> ("Value"=w269:bool)  [unwired: 1 in, 2 out]
        n136 = case shown="真" w269 {
          frame False {
            n137 = One Button Dialog(message="启动失败，请先通电" ("消息")) -> ()  [unwired: 1 in, 1 out]
          }
          frame True {
            n138 = call "多参数传感器参数读取.vi"() -> ("error out"=w272:errorcluster, "添加的数组"=w273:string[][])  [unwired: 10 in]
            n139 = call <vilib>:"General Error Handler.vi"("error in (no error)"=w272) -> ()  [unwired: 10 in, 5 out]
            n140 = property on="传感器区" class="MCListbox (严格)"("ItemNames"=w273) -> ()  [unwired: 2 in, 2 out]
          }
        }
      }
      event "关键参数区读取": Value Change {
        n141 = event-data() -> ()  [unwired: 1 in, 6 out]
        n142 = property class="Bool (严格)"(reference=w275) -> ("Value"=w274:bool)  [unwired: 1 in, 2 out]
        n143 = case shown="假" w274 {
          frame False {
            n144 = One Button Dialog(message="启动失败，请先通电" ("消息")) -> ()  [unwired: 1 in, 1 out]
          }
          frame True {
            n145 = call "多参数关键参数读取.vi"() -> ("error out"=w277:errorcluster, "添加的数组"=w278:string[][])  [unwired: 10 in]
            n146 = call <vilib>:"General Error Handler.vi"("error in (no error)"=w277) -> ()  [unwired: 10 in, 5 out]
            n147 = property on="关键参数区" class="MCListbox (严格)"("ItemNames"=w278) -> ()  [unwired: 2 in, 2 out]
          }
        }
      }
      event "测量数据区读取": Value Change {
        n148 = event-data() -> ()  [unwired: 1 in, 6 out]
        n149 = property class="Bool (严格)"(reference=w280) -> ("Value"=w279:bool)  [unwired: 1 in, 2 out]
        n150 = case shown="假" w279 {
          frame False {
            n151 = One Button Dialog(message="启动失败，请先通电" ("消息")) -> ()  [unwired: 1 in, 1 out]
          }
          frame True {
            n152 = call "多参数测量数据读取.vi"("探头选择"="探头选择") -> ("error out"=w283:errorcluster, "添加的数组"=w284:string[][])  [unwired: 8 in, 1 out]
            n153 = call <vilib>:"General Error Handler.vi"("error in (no error)"=w283) -> ()  [unwired: 10 in, 5 out]
            n154 = property on="测量数据区" class="MCListbox (严格)"("ItemNames"=w284) -> ()  [unwired: 2 in, 2 out]
          }
        }
      }
      event "状态告警区读取": Value Change {
        n155 = event-data() -> ()  [unwired: 1 in, 6 out]
        n156 = property class="Bool (严格)"(reference=w286) -> ("Value"=w285:bool)  [unwired: 1 in, 2 out]
        n157 = case shown="真" w285 {
          frame False {
            n158 = One Button Dialog(message="启动失败，请先通电" ("消息")) -> ()  [unwired: 1 in, 1 out]
          }
          frame True {
            n159 = call "多参数状态告警区读取.vi"() -> ("error out"=w288:errorcluster, "添加的数组"=w289:string[][])  [unwired: 9 in, 1 out]
            n160 = call <vilib>:"General Error Handler.vi"("error in (no error)"=w288) -> ()  [unwired: 10 in, 5 out]
            n161 = property on="状态告警区" class="MCListbox (严格)"("ItemNames"=w289) -> ()  [unwired: 2 in, 2 out]
          }
        }
      }
      event "同步时间": Value Change {
        n162 = event-data() -> ()  [unwired: 1 in, 6 out]
        n163 = property class="Bool (严格)"(reference=w291) -> ("Value"=w290:bool)  [unwired: 1 in, 2 out]
        n164 = case shown="假" w290 {
          frame False {
            n165 = One Button Dialog(message="启动失败，请先通电" ("消息")) -> ()  [unwired: 1 in, 1 out]
          }
          frame True {
            w293 = u16 13 items=["启动测量（全部）"=1, "初始化（清洗）"=10, "停止测量（全部）"=11, "校时"=13, "启动测量（单个传感器）"=19, "停止测量（单个传感器）"=20] ("控制命令")
            w294 = u16 9 items=["氨氮"=3, "水温"=9, "pH值"=10, "溶解氧"=11, "电导率"=12, "浊度"=13, "叶绿素a"=14, "藻密度"=15, "蓝绿藻"=16, "氧化还原电位"=17, "溶解氧%"=18, "盐度"=19] ("站号")
            n166 = call "多参数控制命令.vi"("控制命令"=w293, "站号"=w294) -> ("error out"=w296:errorcluster)  [unwired: 9 in]
            n167 = case shown="错误" w296 {
              tunnel: ["时间同步成功" ("消息") "时间同步失败" ("消息")] -> w295
              frame No Error {
              }
              frame Error {
              }
            }
            n168 = One Button Dialog(message=w295) -> ()  [unwired: 1 in, 1 out]
          }
        }
      }
      event "启动测量(全部)": Value Change {
        n169 = event-data() -> ()  [unwired: 1 in, 6 out]
        n170 = property class="Bool (严格)"(reference=w300) -> ("Value"=w299:bool)  [unwired: 1 in, 2 out]
        n171 = case shown="假" w299 {
          frame False {
            n172 = One Button Dialog(message="启动失败，请先通电" ("消息")) -> ()  [unwired: 1 in, 1 out]
          }
          frame True {
            w302 = u16 1 items=["启动测量（全部）"=1, "初始化（清洗）"=10, "停止测量（全部）"=11, "校时"=13, "启动测量（单个传感器）"=19, "停止测量（单个传感器）"=20] ("控制命令")
            w303 = u16 9 items=["氨氮"=3, "水温"=9, "pH值"=10, "溶解氧"=11, "电导率"=12, "浊度"=13, "叶绿素a"=14, "藻密度"=15, "蓝绿藻"=16, "氧化还原电位"=17, "溶解氧%"=18, "盐度"=19] ("站号")
            n173 = call "多参数控制命令.vi"("控制命令"=w302, "站号"=w303) -> ("error out"=w305:errorcluster)  [unwired: 9 in]
            n174 = case shown="无错误" w305 {
              tunnel: ["启动成功" ("消息") "启动失败" ("消息")] -> w304
              frame No Error {
              }
              frame Error {
              }
            }
            n175 = One Button Dialog(message=w304) -> ()  [unwired: 1 in, 1 out]
          }
        }
      }
      event "停止测量(全部)": Value Change {
        n176 = event-data() -> ()  [unwired: 1 in, 6 out]
        n177 = property class="Bool (严格)"(reference=w309) -> ("Value"=w308:bool)  [unwired: 1 in, 2 out]
        n178 = case shown="真" w308 {
          frame False {
            n179 = One Button Dialog(message="启动失败，请先通电" ("消息")) -> ()  [unwired: 1 in, 1 out]
          }
          frame True {
            w313 = u16 11 items=["启动测量（全部）"=1, "初始化（清洗）"=10, "停止测量（全部）"=11, "校时"=13, "启动测量（单个传感器）"=19, "停止测量（单个传感器）"=20] ("控制命令")
            w314 = u16 9 items=["氨氮"=3, "水温"=9, "pH值"=10, "溶解氧"=11, "电导率"=12, "浊度"=13, "叶绿素a"=14, "藻密度"=15, "蓝绿藻"=16, "氧化还原电位"=17, "溶解氧%"=18, "盐度"=19] ("站号")
            n180 = call "多参数控制命令.vi"("控制命令"=w313, "站号"=w314) -> ("error out"=w312:errorcluster)  [unwired: 9 in]
            n181 = case shown="错误" w312 {
              tunnel: ["停止成功" ("消息") "停止失败" ("消息")] -> w311
              frame No Error {
              }
              frame Error {
              }
            }
            n182 = One Button Dialog(message=w311) -> ()  [unwired: 1 in, 1 out]
          }
        }
      }
      event "初始化(清洗)": Value Change {
        n183 = event-data() -> ()  [unwired: 1 in, 6 out]
        n184 = property class="Bool (严格)"(reference=w318) -> ("Value"=w317:bool)  [unwired: 1 in, 2 out]
        n185 = case shown="真" w317 {
          frame False {
            n186 = One Button Dialog(message="启动失败，请先通电" ("消息")) -> ()  [unwired: 1 in, 1 out]
          }
          frame True {
            w322 = u16 10 items=["启动测量（全部）"=1, "初始化（清洗）"=10, "停止测量（全部）"=11, "校时"=13, "启动测量（单个传感器）"=19, "停止测量（单个传感器）"=20] ("控制命令")
            w323 = u16 9 items=["氨氮"=3, "水温"=9, "pH值"=10, "溶解氧"=11, "电导率"=12, "浊度"=13, "叶绿素a"=14, "藻密度"=15, "蓝绿藻"=16, "氧化还原电位"=17, "溶解氧%"=18, "盐度"=19] ("站号")
            n187 = call "多参数控制命令.vi"("控制命令"=w322, "站号"=w323) -> ("error out"=w320:errorcluster)  [unwired: 9 in]
            n188 = case shown="错误" w320 {
              tunnel: ["初始化成功" ("消息") "初始化失败" ("消息")] -> w321
              frame No Error {
              }
              frame Error {
              }
            }
            n189 = One Button Dialog(message=w321) -> ()  [unwired: 1 in, 1 out]
          }
        }
      }
      event "启动测量(单探)": Value Change {
        n190 = event-data() -> ()  [unwired: 1 in, 6 out]
        n191 = property class="Bool (严格)"(reference=w327) -> ("Value"=w326:bool)  [unwired: 1 in, 2 out]
        n192 = property class="Ring (严格)"(reference=w329) -> ("Value"=w328:u16)  [unwired: 1 in, 2 out]
        n193 = case shown="真" w326 {
          tunnel: w328 -> [_ w331]
          frame False {
            n194 = One Button Dialog(message="启动失败，请先通电" ("消息")) -> ()  [unwired: 1 in, 1 out]
          }
          frame True {
            w332 = u16 19 items=["启动测量（全部）"=1, "初始化（清洗）"=10, "停止测量（全部）"=11, "校时"=13, "启动测量（单个传感器）"=19, "停止测量（单个传感器）"=20] ("控制命令")
            n195 = call "多参数控制命令.vi"("控制命令"=w332, "站号"=w331) -> ("error out"=w334:errorcluster)  [unwired: 9 in]
            n196 = case shown="无错误" w334 {
              tunnel: ["启动成功" ("消息") "启动失败" ("消息")] -> w333
              frame No Error {
              }
              frame Error {
              }
            }
            n197 = One Button Dialog(message=w333) -> ()  [unwired: 1 in, 1 out]
          }
        }
      }
      event "停止测量(单探)": Value Change {
        n198 = event-data() -> ()  [unwired: 1 in, 6 out]
        n199 = property class="Bool (严格)"(reference=w338) -> ("Value"=w337:bool)  [unwired: 1 in, 2 out]
        n200 = property class="Ring (严格)"(reference=w340) -> ("Value"=w339:u16)  [unwired: 1 in, 2 out]
        n201 = case shown="真" w337 {
          tunnel: w339 -> [_ w342]
          frame False {
            n202 = One Button Dialog(message="启动失败，请先通电" ("消息")) -> ()  [unwired: 1 in, 1 out]
          }
          frame True {
            w343 = u16 20 items=["启动测量（全部）"=1, "初始化（清洗）"=10, "停止测量（全部）"=11, "校时"=13, "启动测量（单个传感器）"=19, "停止测量（单个传感器）"=20] ("控制命令")
            n203 = call "多参数控制命令.vi"("控制命令"=w343, "站号"=w342) -> ("error out"=w345:errorcluster)  [unwired: 9 in]
            n204 = case shown="错误" w345 {
              tunnel: ["停止成功" ("消息") "停止失败" ("消息")] -> w344
              frame No Error {
              }
              frame Error {
              }
            }
            n205 = One Button Dialog(message=w344) -> ()  [unwired: 1 in, 1 out]
          }
        }
      }
      event "写入KB": Value Change {
        n206 = event-data() -> ()  [unwired: 1 in, 6 out]
        n207 = property class="DigNum (严格)"(reference=w351) -> ("Value"=w350:dbl)  [unwired: 1 in, 2 out]
        n208 = property class="DigNum (严格)"(reference=w353) -> ("Value"=w352:dbl)  [unwired: 1 in, 2 out]
        n209 = property class="Bool (严格)"(reference=w349) -> ("Value"=w348:bool)  [unwired: 1 in, 2 out]
        n210 = property class="Ring (严格)"(reference=w355) -> ("Value"=w354:u16)  [unwired: 1 in, 2 out]
        n211 = case shown="假" w348 {
          tunnel: w354 -> [_ w361]
          tunnel: w352 -> [_ w360]
          tunnel: w350 -> [_ w359]
          frame False {
            n212 = One Button Dialog(message="启动失败，请先通电" ("消息")) -> ()  [unwired: 1 in, 1 out]
          }
          frame True {
            n213 = call "多参数校准写入.vi"("B"=w360, "K"=w359, "站号"=w361) -> ("error out"=w357:errorcluster)  [unwired: 8 in]
            n214 = case shown="错误" w357 {
              tunnel: ["写入成功" ("消息") "写入失败" ("消息")] -> w358
              frame No Error {
              }
              frame Error {
              }
            }
            n215 = One Button Dialog(message=w358) -> ()  [unwired: 1 in, 1 out]
          }
        }
      }
      event "K", "B": Mouse Down {
        n216 = event-data() -> ("CtlRef"=w367:refnum<vi>)  [unwired: 1 in, 5 out]
        n217 = property class="DigNum (严格)"(reference=w367) -> (reference out=w366:refnum<vi>, "Value"=w365:dbl)  [unwired: 1 in, 1 out]
        n218 = call "数字键盘.vi"("OldNumber"=w365) -> ("NewNumber"=w364:sgl)
        n219 = property class="DigNum (严格)"(reference=w366, "Value"=w364) -> ()  [unwired: 1 in, 2 out]
      }
      event "读取KB": Value Change {
        n220 = event-data() -> ()  [unwired: 1 in, 6 out]
        n221 = property class="Bool (严格)"(reference=w369) -> ("Value"=w368:bool)  [unwired: 1 in, 2 out]
        n222 = property class="Ring (严格)"(reference=w371) -> ("Value"=w370:u16)  [unwired: 1 in, 2 out]
        n223 = case shown="真" w368 {
          tunnel: w370 -> [_ w375]
          frame False {
            n224 = One Button Dialog(message="启动失败，请先通电" ("消息")) -> ()  [unwired: 1 in, 1 out]
          }
          frame True {
            n225 = call "多参校准读取.vi"("站号"=w375) -> ("error out"=w373:errorcluster, "B"=→"B":dbl, "K"=→"K":dbl)  [unwired: 8 in]
            n226 = case shown="无错误" w373 {
              tunnel: ["读取成功" ("消息") "读取失败" ("消息")] -> w374
              frame No Error {
              }
              frame Error {
              }
            }
            n227 = One Button Dialog(message=w374) -> ()  [unwired: 1 in, 1 out]
          }
        }
      }
      event "自动校准": Value Change {
        n228 = event-data() -> ()  [unwired: 1 in, 6 out]
        n229 = property class="Bool (严格)"(reference=w381) -> ("Value"=w380:bool)  [unwired: 1 in, 2 out]
        n230 = case shown="真" w380 {
          frame False {
            n231 = One Button Dialog(message="启动失败，请先通电" ("消息")) -> ()  [unwired: 1 in, 1 out]
          }
          frame True {
            n232 = call "多参校准.vi"() -> ()  [unwired: 12 in]
          }
        }
      }
      event "手动通电": Value Change {
        n233 = event-data() -> ("NewVal"=w384:bool)  [unwired: 1 in, 5 out]
        n234 = Boolean To (0,1)(Boolean=w384) -> (0, 1=w383:i16)
        n235 = Bundle By Name(cluster=T9 {"starting address"=0, "holding register value"=0}, "starting address"=u16 302, "holding register value"=w383) -> (w386:T9)
        n236 = call "采配水通讯指令.vi"("数据"=w386, "命令"=T10."单个写入") -> ()  [unwired: 10 in]
      }
    }
  }
